vi "Serial_Arduino.vi"() -> ()   [LabVIEW 2017]
doc: "This example performs writes and reads on a serial port, as directed by the user. You can press the Write and Read buttons, and change the Read Count, while the example is running.\n\nThe parameters set for the serial port must match the parameters of the connected instrument or device. In this example, the Read Count parameter specifies the number of bytes that the serial port reads. If there were more bytes at the port than the specified number, those bytes would not be read. If there were less bytes at the port than the specified number, you would receive a timeout error.\n\nThis example expands upon the flow control options for XON and XOFF, allowing the user to choose those control characters. Also, the user can enable or disable a termination character. Some devices require a termination character in order to identify the end of command strings. Some devices send a termination character to signify the end of data to be read. This example shows how you can end the Read operation once a termination character is detected in the buffer and/or append a termination character at the end of the Write data."
uses:
  <vilib>/Instr/_visa.llb/VISA Configure Serial Port (Instr).vi
panel:
  out "Tangaj":dbl(graph)
  out "Ruliu":dbl(graph)
  in  "baud rate (9600)":u32=9600
  out "Z":dbl(graph)
  out "Y":dbl(graph)
  out "X":dbl(graph)=-207.0
  in  "Stop":bool
  in  "Read Count":u32=1000
  out "Serial":string
  in  "START":bool
  in  "Port":refnum<visa-resource-name>="COM1"
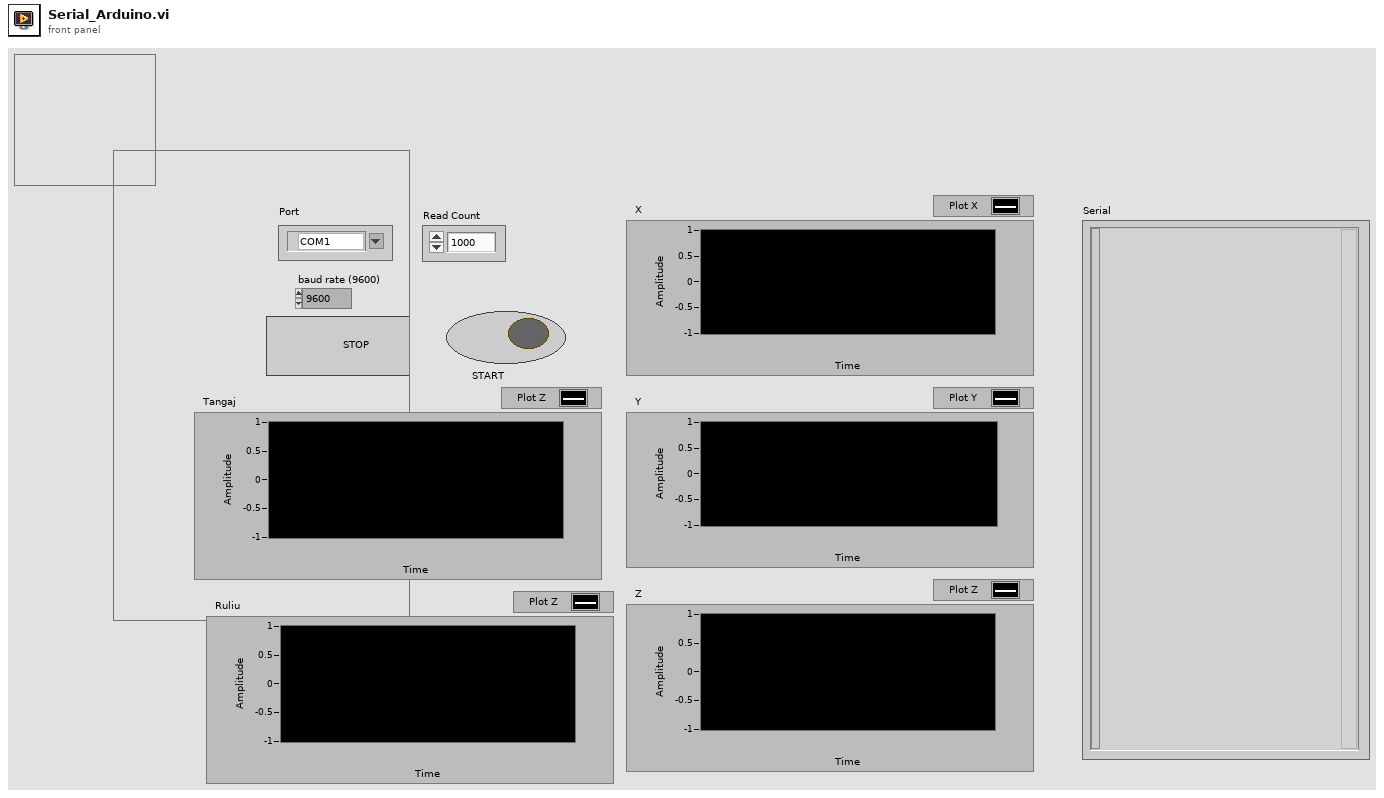
[diagram p1: front panel]
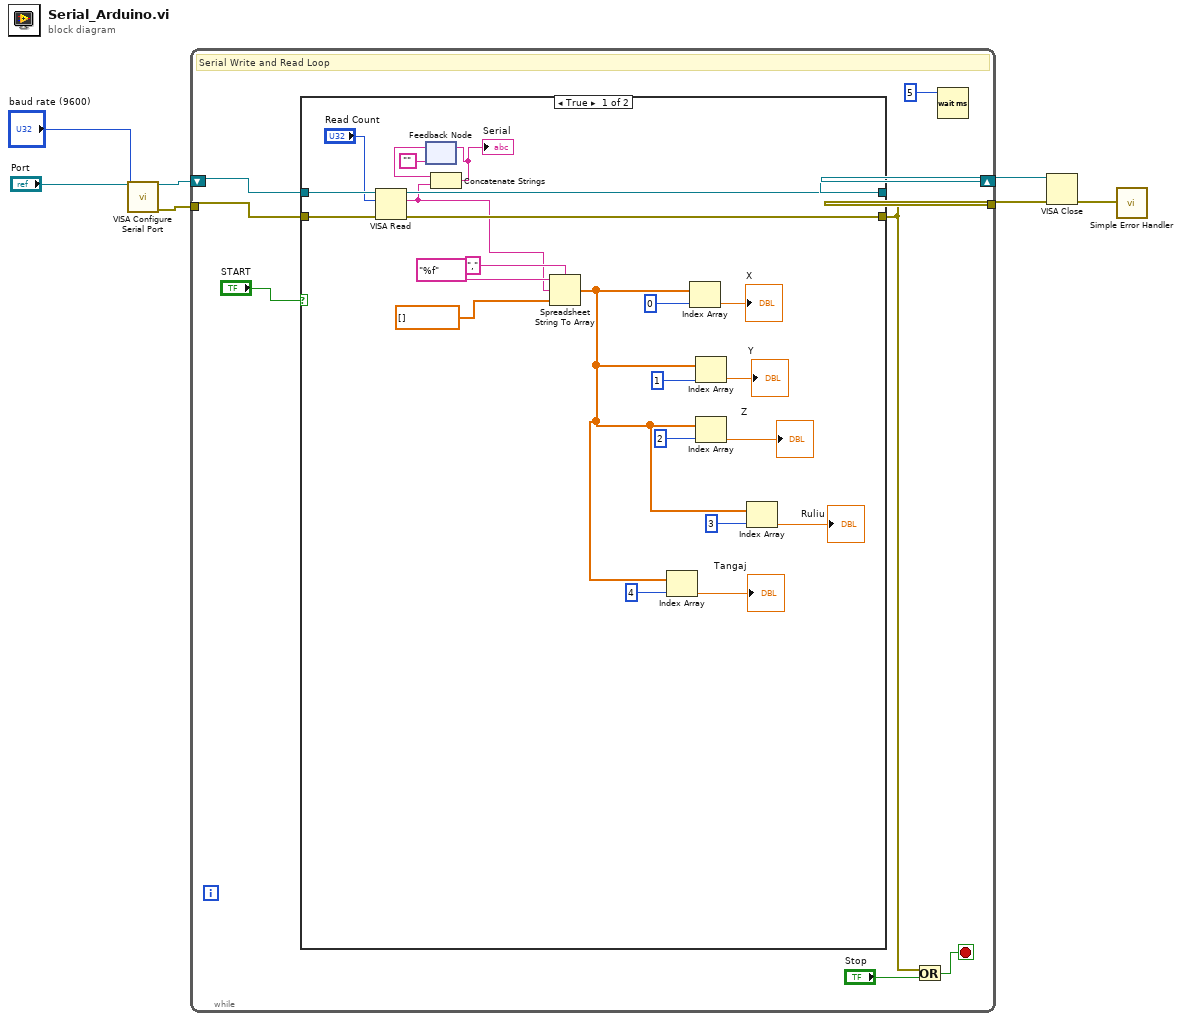
[diagram p0: block diagram]
diagram:
  n1 = call-poly "VISA Configure Serial Port"("VISA resource name"="Port", "baud rate (9600)"="baud rate (9600)") -> ("VISA resource name out"=w3:refnum<visa-resource-name>, "error out"=w2:errorcluster)  [unwired: 8 in, 4 out]
  n2 = while {
    shift-right: [w15] -> w4
    shift-left: w3 -> [w12]
    tunnel: w2 -> [w11]
    tunnel: [w13] -> w5
    stop <- w8 stop-if-true
    # "Serial Write and Read Loop"
    n3 = case shown="True" "START" {
      tunnel: [w36 w40] -> w15
      tunnel: w12 -> [w38 w40]
      tunnel: [w34 w39] -> w13
      tunnel: w11 -> [w37 w39]
      frame True {
        n4 = VISA Read(VISA resource name=w38, byte count="Read Count", error in (no error)=w37) -> (VISA resource name out=w36:refnum<visa-resource-name>, read buffer=w27:string, error out=w34:errorcluster)  [unwired: 1 out]
        n5 = feedback #1("") -> (w33:string)
        n6 = Concatenate Strings(w33, w27) -> (w28:string)
        "Serial" <- w28
        n7 = feedback-in #1(w28) -> ()
        n8 = Spreadsheet String To Array(delimiter (Tab)=",", format string="%f", spreadsheet string=w27, array type (2D Dbl)=dbl[] [] ("Data Graph")) -> (array=w16:dbl[])
        n9 = Index Array(array=w16, index=4 ("disabled index (col)")) -> (element=→"Tangaj":dbl)
        n10 = Index Array(array=w16, index=0 ("disabled index (col)")) -> (element=→"X":dbl)
        n11 = Index Array(array=w16, index=1 ("disabled index (col)")) -> (element=→"Y":dbl)
        n12 = Index Array(array=w16, index=2 ("disabled index (col)")) -> (element=→"Z":dbl)
        n13 = Index Array(array=w16, index=3 ("disabled index (col)")) -> (element=→"Ruliu":dbl)
      }
      frame False {
      }
    }
    n14 = Or(x=w13, y="Stop") -> (x .or. y?=w8:bool)
    n15 = Wait (ms)(milliseconds to wait=u32 5) -> ()  [unwired: 1 out]
  }
  n16 = VISA Close(VISA resource name=w4, error in (no error)=w5) -> (error out=w6:errorcluster)
  n17 = call <vilib>:"Simple Error Handler.vi"("error in (no error)"=w6) -> ()  [unwired: 1 in, 8 out]
